vi "Passwort loeschen.vi"(10 "Passworte":T1) -> (2 "Passworte":T1)   [LabVIEW 2020, in "Passwort.lvlib"]
uses:
  Passwort.lvlib
  Passwort Array.ctl
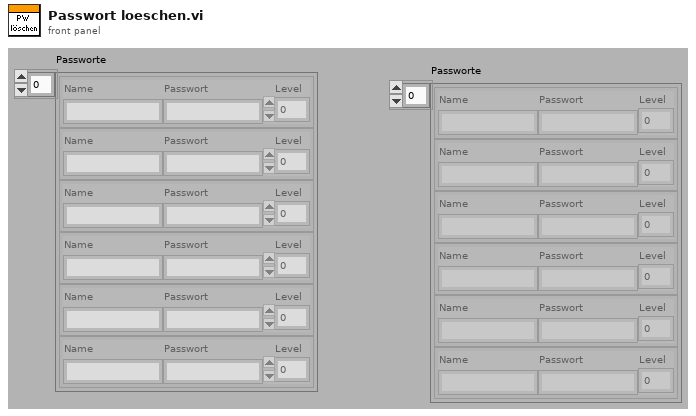
[diagram p1: front panel]
types:
  T1 = typedef "Passwort.lvlib/Passwort Array.ctl" = cluster{"Name":string, "Passwort":string, "Level":i16}[]
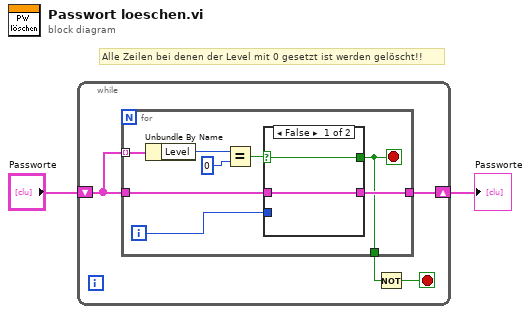
[diagram p0: block diagram]
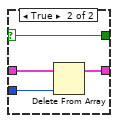
[diagram p2: hidden frame]
diagram:
  # "Alle Zeilen bei denen der Level mit 0 gesetzt ist werden gelöscht!!"
  n1 = while {
    shift-right: [w5] -> w1
    shift-left: "Passworte" -> [w6]
    stop <- w3 stop-if-true
    n2 = for {
      tunnel: w6 -> [w10] mode=indexing
      tunnel: w6 -> [w9]
      tunnel: [w8] -> w5
      tunnel: [w7] -> w4
      i -> [w12]
      stop <- w7 stop-if-true
      n3 = Unbundle By Name(w10) -> ("Level"=w14:i16)
      n4 = Equal?(x=w14, y=i16 0) -> (x = y?=w11:bool)
      n5 = case shown="False" w11 {
        selector: w11 -> [w15 w17]
        tunnel: w12 -> [_ w19]
        tunnel: w9 -> [w16 w20]
        tunnel: [w16 w18] -> w8
        tunnel: [w15 w17] -> w7
        frame False {
        }
        frame True {
          n6 = Delete From Array(array=w20, index=w19) -> (array with subset deleted=w18:T1)  [unwired: 1 in, 1 out]
        }
      }
    }
    n7 = Not(x=w4) -> (.not. x?=w3:bool)
  }
  "Passworte" <- w1
